vi "Init_DAQ_AO.vi"(8 "error in":errorcluster, 11 "Prueba31 in":refnum<class "Prueba33.lvclass">) -> (0 "error out":errorcluster, 3 "Prueba31 out":refnum<class "Prueba33.lvclass">)   [LabVIEW 2019, in "Prueba33.lvclass"]
uses:
  Prueba33.lvclass
  Prueba33.lvclass/Prueba33.ctl
  <vilib>/DAQmx/write.llb/DAQmx Write (Analog 1D Wfm NChan NSamp).vi
  <vilib>/DAQmx/create/channels.llb/DAQmx Create Channel (AO-Voltage-Basic).vi
  <vilib>/DAQmx/configure/timing.llb/DAQmx Timing (Sample Clock).vi
  <vilib>/DAQmx/miscellaneous.llb/DAQmx Fill In Error Info.vi
  <vilib>/measure/NI_MABase.lvlib
panel:
  in  "AO Array":T1(array[cluster])=[{"Waveform Type"=0, "Amplitude"=0.0, "Frequency"=0.0}, {"Waveform Type"=0, "Amplitude"=0.0, "Frequency"=0.0}, {"Waveform Type"=0, "Amplitude"=0.0, "Frequency"=0.0}, {"Waveform Type"=0, "Amplitude"=0.0, "Frequency"=0.0}] {"Frequency" format="%0.2p"; "Amplitude" format="%0.2p"; "Waveform Type" items=["Sine Wave", "Triangle Wave", "Square Wave", "Sawtooth Wave"]}
  # "AO0"
  # "AO1"
  # "AO2"
  # "AO3"
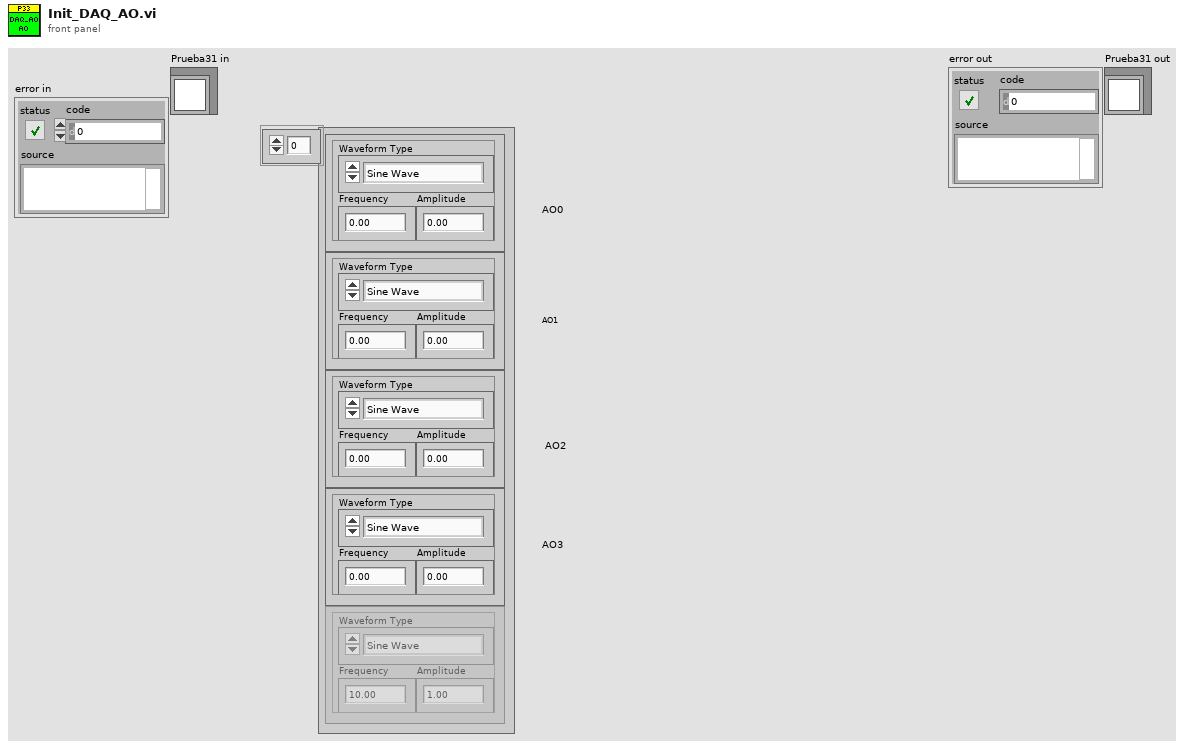
[diagram p1: front panel]
types:
  T1 = cluster{"Waveform Type":u16, "Amplitude":dbl, "Frequency":dbl}[]
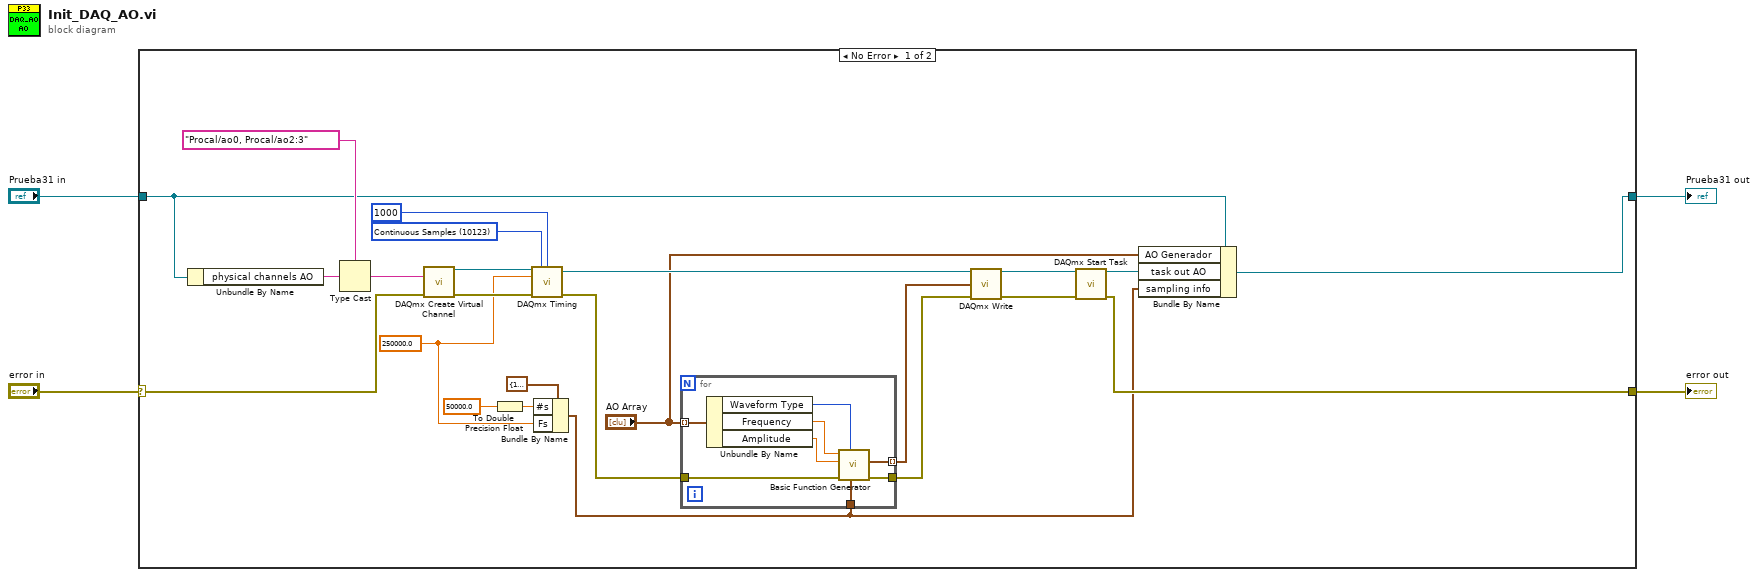
[diagram p0: block diagram]
diagram:
  n1 = case shown="No Error" "error in" {
    selector: "error in" -> [w8 w38]
    tunnel: [w7 w38] -> w3
    tunnel: [w10 w37] -> w2
    tunnel: "Prueba31 in" -> [w9 w37]
    frame No Error {
      w17 = 250000.0 ("rate")
      w22 = 10123 items=["Finite Samples"=10178, "Continuous Samples"=10123, "Hardware Timed Single Point"=12522] ("sample mode")
      n2 = Unbundle By Name(w9) -> ("physical channels AO"=w27:string)
      n3 = Type Cast(type=tag "Procal/ao0, Procal/ao2:3" ("physical channels"), x=w27) -> (*(type *) &x=w26:tag)
      n4 = call-poly <vilib>:"DAQmx Create Virtual Channel.vi"("physical channels"=w26, "error in"=w8) -> ("task out"=w24:refnum<k21>, "error out"=w25:errorcluster)  [unwired: 12 in]
      n5 = To Double Precision Float(number=50000.0) -> (double precision float=w19:dbl)
      n6 = call-poly <vilib>:"DAQmx Timing.vi"("task/channels in"=w24, "sample mode"=w22, "samples per channel"=1000, "rate"=w17, "error in"=w25) -> ("task out"=w15:refnum<k21>, "error out"=w21:errorcluster)  [unwired: 9 in]
      n7 = Bundle By Name(cluster=cluster{"Fs":dbl, "#s":dbl} {"Fs"=1000.0, "#s"=1000.0} ("sampling info"), "#s"=w19, "Fs"=w17) -> (w5:cluster{"Fs":dbl, "#s":dbl})
      n8 = for {
        tunnel: w5 -> [w36]
        tunnel: "AO Array" -> [w35] mode=indexing
        tunnel: [w31] -> w14 mode=indexing
        tunnel: w21 -> [w30]
        tunnel: [w29] -> w16
        n9 = Unbundle By Name(w35) -> ("Waveform Type"=w34:u16, "Frequency"=w33:dbl, "Amplitude"=w32:dbl)
        n10 = call <vilib>:"Basic Function Generator.vi"("sampling info"=w36, "signal type"=w34, "error in (no error)"=w30, "amplitude"=w32, "frequency"=w33) -> ("error out"=w29:errorcluster, "signal out"=w31:waveform(dbl))  [unwired: 4 in, 1 out]
      }
      n11 = call-poly <vilib>:"DAQmx Write.vi"("task/channels in"=w15, "data"=w14, "error in"=w16) -> ("task out"=w12:refnum<k21>, "error out"=w13:errorcluster)  [unwired: 10 in, 1 out]
      n12 = call <vilib>:"DAQmx Start Task.vi"("task/channels in"=w12, "error in"=w13) -> ("task out"=w11:refnum<k21>, "error out"=w7:errorcluster)  [unwired: 12 in]
      n13 = Bundle By Name(cluster=w9, "AO Generador"="AO Array", "task out AO"=w11, "sampling info"=w5) -> (w10:refnum<class "Prueba33.lvclass">)
    }
    frame Error {
    }
  }
  "error out" <- w3
  "Prueba31 out" <- w2
